vi "Untitled 1 (SubVI).vi"(11 "string":string) -> (3 "number":u32)   [LabVIEW 2015]
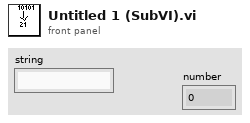
[diagram p1: front panel]
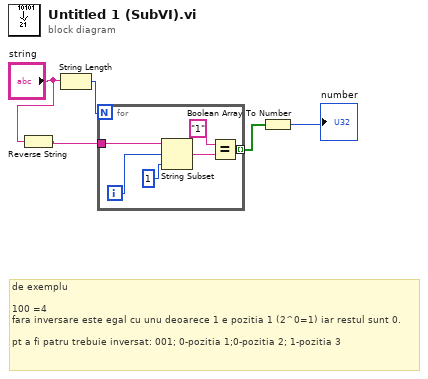
[diagram p0: block diagram]
diagram:
  # "de exemplu \n\n100 =4 \nfara inversare este egal cu unu deoarece 1 e pozitia 1 (2^0=1) iar restul sunt 0.\n\npt a fi patru trebuie inversat: 001; 0-pozitia 1;0-pozitia 2; 1-pozitia 3"
  n1 = Reverse String(1:"string") -> (0:w1:string)
  n2 = String Length(string="string") -> (length=w5:i32)
  n3 = for {
    N: w5 -> [_]
    tunnel: [w7] -> w4 mode=indexing
    tunnel: w1 -> [w6]
    i -> [w10]
    n4 = String Subset(string=w6, offset (0)=w10, length (rest)=1 ("length (rest)")) -> (substring=w9:string)
    n5 = Equal?(x="1", y=w9) -> (x = y?=w7:bool)
  }
  n6 = Boolean Array To Number(Boolean array=w4) -> (number=→"number":u32)
